vi "De-Initialize.vi"(8 "error in (no error)":errorcluster, 11 "Tektronix MSO 6 Driver in":refnum<class "Tektronix MSO 6 Driver.lvclass">) -> (0 "error out":errorcluster, 3 "Tektronix MSO 6 Driver out":refnum<class "Tektronix MSO 6 Driver.lvclass">)   [LabVIEW 2020, in "Tektronix MSO 6 Driver.lvclass"]
uses:
  Tektronix MSO 6 Driver.lvclass
  C:/GitHub/NHMFL_Core/Libraries/Instruments/Tektronix/Tektronix Driver/Tektronix Driver.lvclass
  <instrlib>/Tektronix MSO5X Series/Tektronix MSO5X Series.lvlib
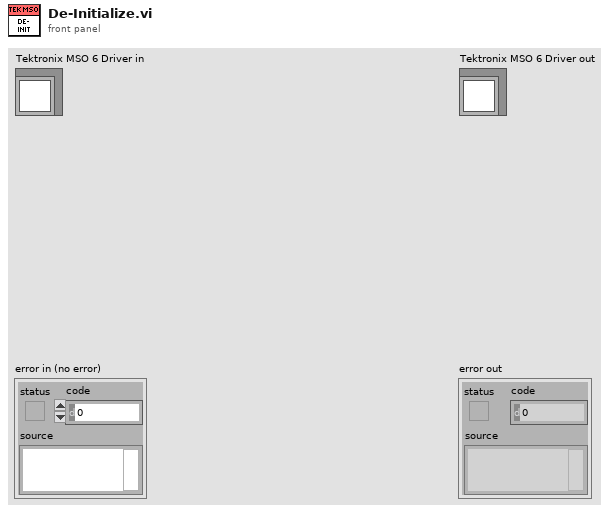
[diagram p1: front panel]
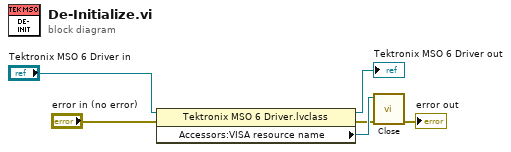
[diagram p0: block diagram]
diagram:
  n1 = property class="Tektronix MSO 6 Driver.lvclass"(reference="Tektronix MSO 6 Driver in", error in="error in (no error)") -> (reference out=→"Tektronix MSO 6 Driver out":refnum<class "Tektronix MSO 6 Driver.lvclass">, error out=w3:errorcluster, "Accessors:VISA resource name"=w5:refnum<visa-resource-name>)
  n2 = call <instrlib>:"Close.vi"("error in (no error)"=w3, "VISA resource name"=w5) -> ("error out"=→"error out":errorcluster)  [unwired: 9 in]
